vi "Display Map Loop.vi"() -> (3 "Intensity Graph":u16[][](graph))   [LabVIEW 2017]
uses:
  Control Globals.vi
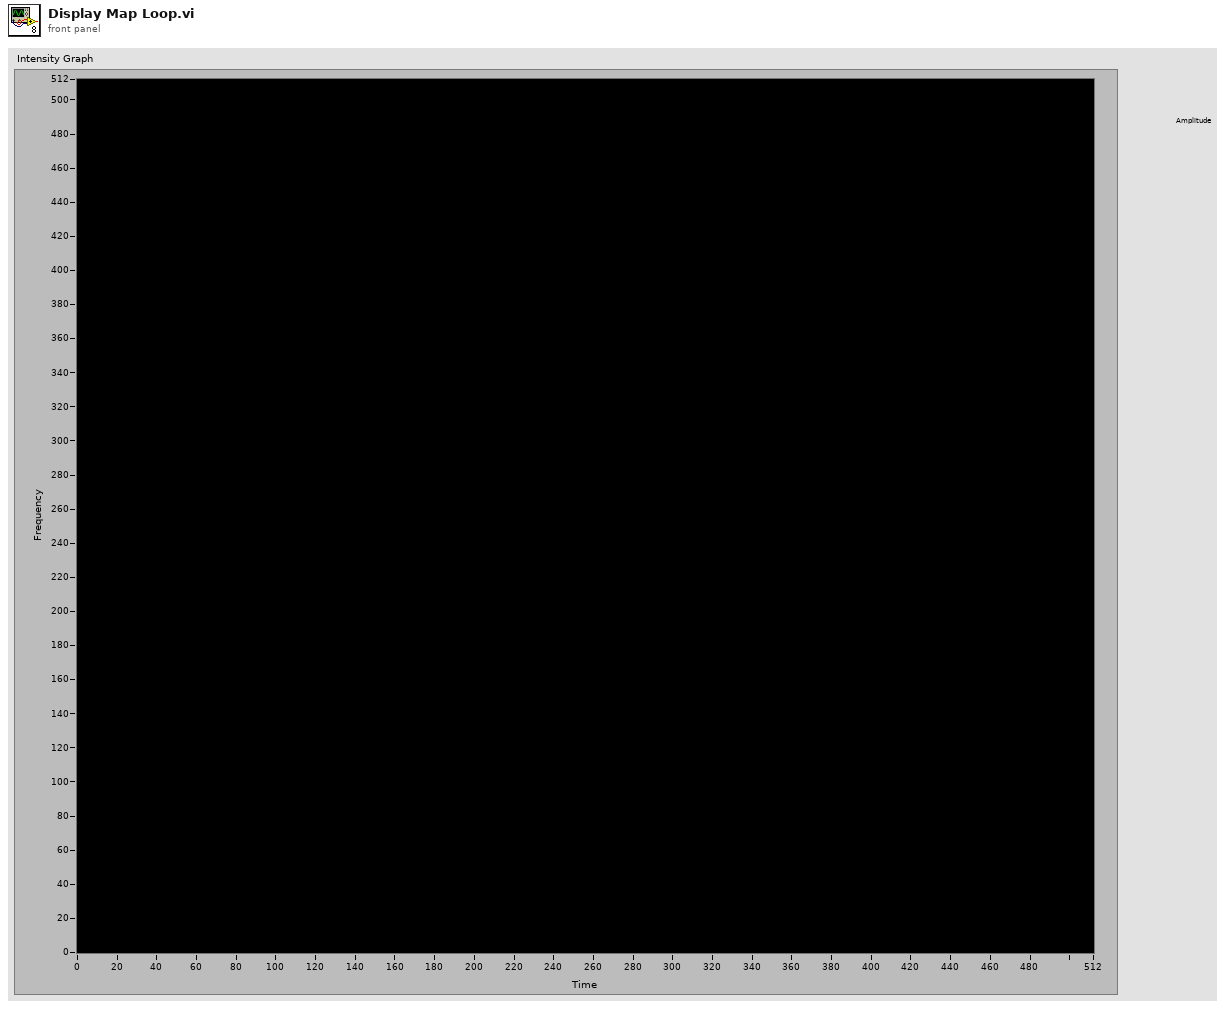
[diagram p1: front panel]
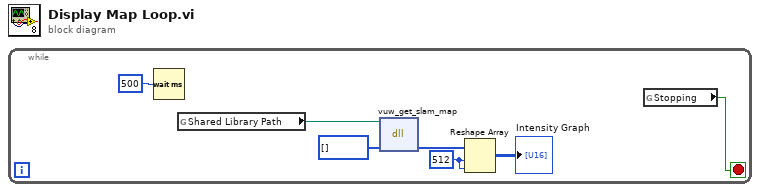
[diagram p0: block diagram]
diagram:
  n1 = while {
    stop <- w2 stop-if-true
    w6 = 512 ("dimension size")
    n2 = Wait (ms)(milliseconds to wait=u32 500) -> ()  [unwired: 1 out]
    n3 = global read "Control Globals.vi" "Shared Library Path"() -> (w1:path)
    n4 = dll-call lib="home/admin/lib/libslam.so" fn="vuw_get_slam_map"(path in=w1, "map"=u16[] []) -> ("map"=w7:u16[])  [unwired: 3 in, 2 out]
    n5 = Reshape Array(w7, w6, w6) -> (→"Intensity Graph":u16[][])
    n6 = global read "Control Globals.vi" "Stopping"() -> (w2:bool)
  }
